vi "mobileyelanepaser3.vi"(8 "thresh  c":dbl, 9 "thresh  b":dbl, 11 "thresh r":dbl) -> (0 "cr2":dbl=0.017, 1 "cr":dbl=1.4, 2 "cl2":dbl=0.017, 3 "cl":dbl=-1.5000000000000002)   [LabVIEW 2015]
uses:
  G_LCM.vi
  G_SEN.vi
panel:
  out "cr_old":dbl
  out "cl_old":dbl
  out "r_old":dbl
  out "t0":i64
  out "b_old":dbl
  out "a2":dbl
  out "b2":dbl=0.017
  out "r2":dbl
  in  "a_cut":dbl=0.01
  out "appended array 2":bool[](array[boolean])=[TRUE, TRUE, FALSE, TRUE, TRUE, FALSE, TRUE]
  out "appended array":dbl[](array[numeric])=[0.65, 0.000478076055664682, 0.04157183092736362, 1.1538500967845816e-15]
  in  "path_gain":dbl=0.95
  in  "q_cut":dbl=0.5
  in  "dc_cut":dbl=0.55
  in  "db_cut":dbl=0.042
  in  "da_cut":dbl=0.0045
  out "lane_old":dbl[](array[numeric])=[0.0006866761302459269, 1.5821018040866166e-06, -1.3046846474672603e-05, 0.0001716690325614815]
  in  "gain":dbl=1.0
  out "dt":dbl=0.096219
  out "count":u64
  out "lane_empty":dbl[](array[numeric])
  out "Lane_R_M":dbl[](array[numeric])=[0.8, 0.0036309999999999997, 0.017, 1.4]
  out "Lane_L_M":dbl[](array[numeric])=[0.8, 0.0036309999999999997, 0.017, -1.5000000000000002]
  out "r":dbl=137.70311209033324
  in  "shift_c":dbl=-0.1
  in  "bias_b":dbl=0.005
  out "a":dbl=0.0036309999999999997
  out "b":dbl=0.017
  out "confidance_L":u8=2
  out "confidance_R":u8=2
  in  "bias_c":dbl=0.8
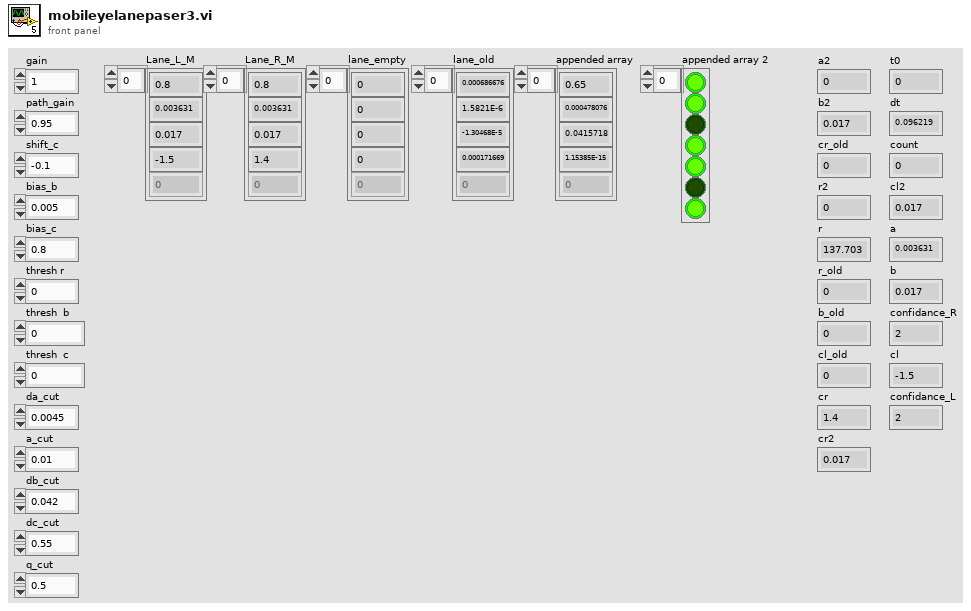
[diagram p1: front panel]
types:
  T1 = cluster{"hash":i64, "sys time":i64, "mobileye":u8[]}
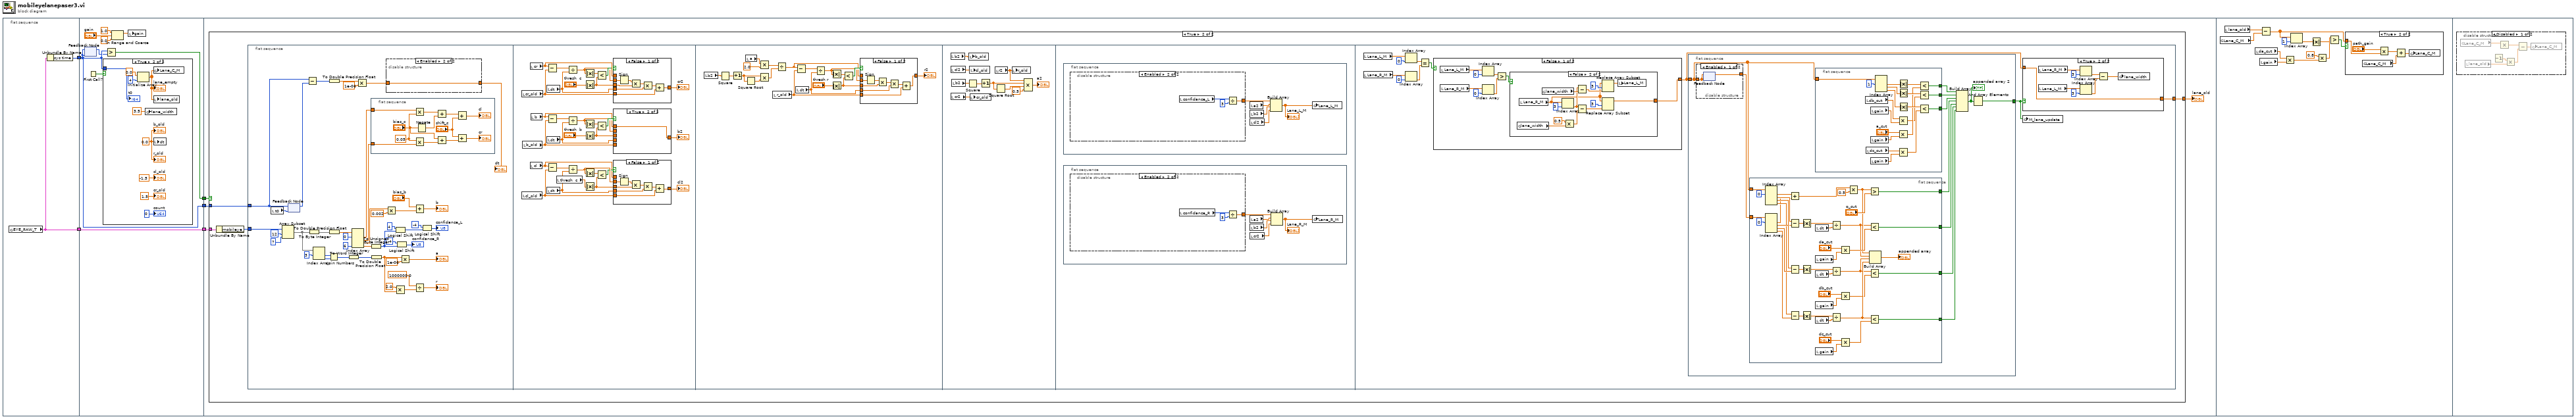
[diagram p0: block diagram]
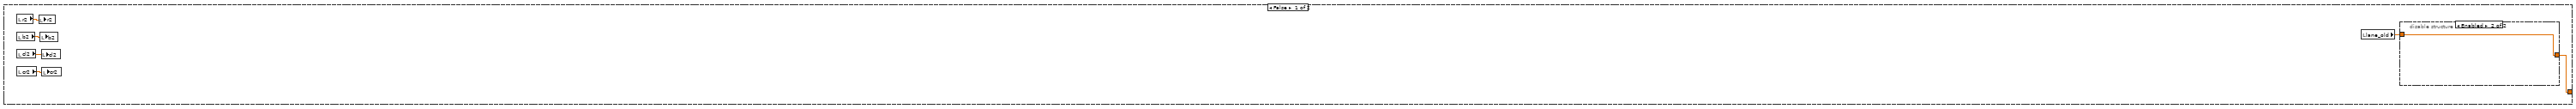
[diagram p3: hidden frame]
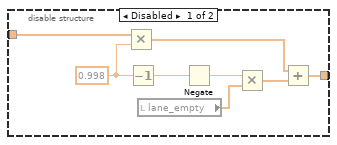
[diagram p4: hidden frame]
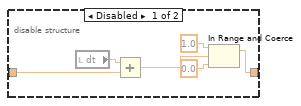
[diagram p5: hidden frame]
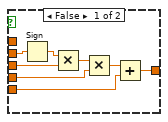
[diagram p8: hidden frame]
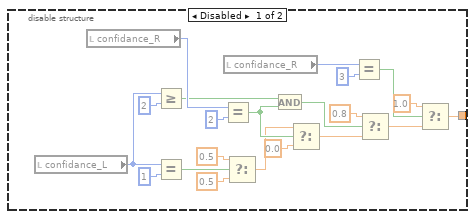
[diagram p10: hidden frame]
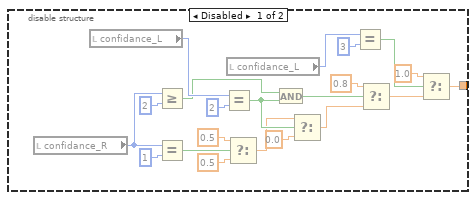
[diagram p11: hidden frame]
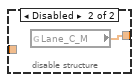
[diagram p12: hidden frame]
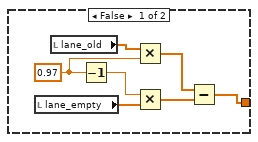
[diagram p13: hidden frame]
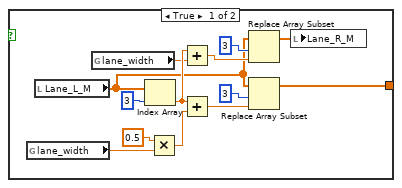
[diagram p14: hidden frame]
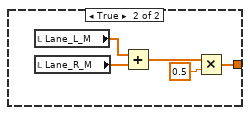
[diagram p15: hidden frame]
diagram:
  n1 = flat-sequence {
    tunnel: [w7] -> w5
    tunnel: [w6] -> w4
    tunnel: w5 -> [w16]
    tunnel: [w16] -> w3
    tunnel: w4 -> [w9]
    tunnel: [w10] -> w2
    tunnel: [w9] -> w1
    tunnel: w3 -> [w29]
    tunnel: w2 -> [w26]
    tunnel: w1 -> [w27]
    frame #0 {
      n2 = global read "G_LCM.vi" "EYE_RAW_T"() -> (w7:T1)
      n3 = Unbundle By Name(w7) -> ("sys time"=w6:i64)
    }
    frame #1 {
      n4 = feedback #1(w9) -> (w8:i64)
      n5 = feedback-in #1(w9) -> ()
      n6 = First Call?() -> (First Call?: T/F=w15:bool)
      n7 = case shown="True" w15 {
        tunnel: w9 -> [_ w20]
        frame False {
        }
        frame True {
          w19 = 0.0 ("dt2")
          n8 = Initialize Array(0.0 ("element"), 4 ("dimension size")) -> (w21:dbl[])
          "lane_empty" <- w21
          n9 = global write "G_SEN.vi" "lane_width"(3.5 ("lane_width")) -> ()
          n10 = global write "G_SEN.vi" "Lane_C_M"(w21) -> ()
          n11 = local write "lane_old"(w21) -> ()
          n12 = local write "dt"(w19) -> ()
          "count" <- u64 0
          "b_old" <- w19
          "t0" <- w20
          "r_old" <- w19
          "cl_old" <- -1.5 ("cl_old")
          "cr_old" <- 1.5 ("cr_old")
        }
      }
      n13 = Greater?(x=w9, y=w8) -> (0:w10:bool)
      n14 = In Range and Coerce(upper limit=1.0, x="gain", lower limit=0.0) -> (coerced(x)=w11:dbl)  [unwired: 1 out]
      n15 = local write "gain"(w11) -> ()
    }
    frame #2 {
      n16 = case shown="True" w26 {
        tunnel: w29 -> [_ w47]
        tunnel: [w34 w46] -> w28
        tunnel: w27 -> [_ w45]
        frame False {
          n17 = local read "r2"() -> (w33:dbl)
          n18 = local read "b2"() -> (w32:dbl)
          n19 = local read "cl2"() -> (w30:dbl)
          n20 = local read "cr2"() -> (w31:dbl)
          n21 = local write "r2"(w33) -> ()
          n22 = local write "b2"(w32) -> ()
          n23 = local write "cl2"(w30) -> ()
          n24 = local write "cr2"(w31) -> ()
          n25 = local read "lane_old"() -> (w35:dbl[])
          n26 = disable-structure shown="Enabled" {
            disable-tunnel: w35 -> [w39 w44]
            disable-tunnel: [w36 w44] -> w34
            frame Disabled {
              w38 = 0.998
              n27 = Multiply(x=w39, y=w38) -> (x*y=w42:dbl[])
              n28 = Decrement(x=w38) -> (x-1=w40:dbl)
              n29 = local read "lane_empty"() -> (w37:dbl[])
              n30 = Negate(x=w40) -> (-x=w41:dbl)
              n31 = Multiply(x=w41, y=w37) -> (x*y=w43:dbl[])
              n32 = Add(x=w42, y=w43) -> (x+y=w36:dbl[])
            }
            frame Enabled {
            }
          }
        }
        frame True {
          n33 = Unbundle By Name(w47) -> ("mobileye"=w48:u8[])
          n34 = flat-sequence {
            tunnel: w48 -> [w69]
            tunnel: w45 -> [w51]
            tunnel: [w264] -> w46
            frame #0 {
              n35 = local read "t0"() -> (w50:i64)
              n36 = Array Subset(array=w69, index=12, length=7) -> (w68:u8[])
              n37 = feedback #2(w50) -> (w52:i64)
              n38 = feedback-in #2(w51) -> ()
              n39 = Subtract(x=w51, y=w52) -> (x-y=w53:i64)
              n40 = To Byte Integer(number=w68) -> (8bit integer=w88:i8[])
              n41 = Index Array(array=w68, index #1=3 ("index")) -> (element #1=w82:u8, element #2=w81:u8)  [unwired: 1 in]
              n42 = Join Numbers(hi=w82, lo=w81) -> ((hi.lo)=w80:u16)
              n43 = To Double Precision Float(number=w53) -> (double precision float=w57:dbl)
              n44 = To Double Precision Float(number=w88) -> (double precision float=w87:dbl[])
              n45 = To Word Integer(number=w80) -> (16bit integer=w79:i16)
              n46 = Index Array(array=w87, index #1=0 ("index"), index #4=6 ("index")) -> (element #1=w86:dbl, element #2=w85:dbl, element #3=w84:dbl, element #4=w75:dbl)  [unwired: 2 in]
              n47 = Multiply(x=w57, y=1e-06) -> (x*y=w55:dbl)
              n48 = To Unsigned Byte Integer(number=w75) -> (unsigned 8bit integer=w73:u8)
              n49 = To Double Precision Float(number=w79) -> (double precision float=w58:dbl)
              n50 = flat-sequence {
                tunnel: w86 -> [w110]
                tunnel: w85 -> [w109]
                frame #0 {
                  w108 = 0.05 ("y")
                  n51 = Multiply(x=w110, y=w108) -> (x*y=w106:dbl)
                  n52 = Multiply(x=w108, y=w109) -> (x*y=w107:dbl)
                  n53 = Negate(x="bias_c") -> (-x=w104:dbl)
                  n54 = Add(x=w106, y=w104) -> (x+y=w103:dbl)
                  n55 = Add(x="bias_c", y=w107) -> (x+y=w101:dbl)
                  n56 = Add(x=w103, y="shift_c") -> (x+y=→"cl":dbl)
                  n57 = Add(x="shift_c", y=w101) -> (x+y=→"cr":dbl)
                }
              }
              n58 = Multiply(x=w84, y=0.002) -> (x*y=w65:dbl)
              n59 = disable-structure shown="Enabled" {
                disable-tunnel: w55 -> [w97 w98]
                disable-tunnel: [w92 w98] -> w54
                frame Disabled {
                  n60 = local read "dt"() -> (w96:dbl)
                  n61 = Add(x=w96, y=w97) -> (x+y=w95:dbl)
                  n62 = In Range and Coerce(upper limit=1.0, x=w95, lower limit=0.0) -> (coerced(x)=w92:dbl)  [unwired: 1 out]
                }
                frame Enabled {
                }
              }
              "dt" <- w54
              n63 = Logical Shift(y=i16 4, x=w73) -> (x << y=w71:u8)
              n64 = Multiply(x=2.0, y=w58) -> (x*y=w61:dbl)
              n65 = Logical Shift(y=i16 -4, x=w73) -> (x << y=→"confidance_R":u8)
              n66 = Multiply(x=w58, y=1e-06) -> (x*y=→"a":dbl)
              n67 = Add(x="bias_b", y=w65) -> (x+y=→"b":dbl)
              n68 = Divide(x=1000000.0 ("y"), y=w61) -> (x/y=→"r":dbl)
              n69 = Logical Shift(y=i16 -4, x=w71) -> (x << y=→"confidance_L":u8)
            }
            frame #1 {
              n70 = local read "cr_old"() -> (w112:dbl)
              n71 = local read "cl_old"() -> (w131:dbl)
              n72 = local read "b_old"() -> (w132:dbl)
              n73 = local read "cr"() -> (w121:dbl)
              n74 = local read "cl"() -> (w123:dbl)
              n75 = local read "b"() -> (w122:dbl)
              n76 = Subtract(x=w121, y=w112) -> (x-y=w119:dbl)
              n77 = Subtract(x=w122, y=w132) -> (x-y=w139:dbl)
              n78 = Subtract(x=w123, y=w131) -> (x-y=w125:dbl)
              n79 = local read "dt"() -> (w113:dbl)
              n80 = local read "dt"() -> (w133:dbl)
              n81 = local read "dt"() -> (w130:dbl)
              n82 = local read "thresh  c"() -> (w111:dbl)
              n83 = Divide(x=w119, y=w113) -> (x/y=w115:dbl)
              n84 = Divide(x=w139, y=w133) -> (x/y=w135:dbl)
              n85 = Divide(x=w125, y=w130) -> (x/y=w128:dbl)
              n86 = Absolute Value(x=w115) -> (abs(x)=w118:dbl)
              n87 = Absolute Value(x="thresh  c") -> (abs(x)=w114:dbl)
              n88 = Absolute Value(x=w135) -> (abs(x)=w138:dbl)
              n89 = Absolute Value(x="thresh  b") -> (abs(x)=w134:dbl)
              n90 = Absolute Value(x=w128) -> (abs(x)=w126:dbl)
              n91 = Absolute Value(x=w111) -> (abs(x)=w129:dbl)
              n92 = Less?(x=w118, y=w114) -> (x < y?=w117:bool)
              n93 = Less?(x=w138, y=w134) -> (x < y?=w137:bool)
              n94 = Less?(x=w126, y=w129) -> (x < y?=w127:bool)
              n95 = case shown="False" w117 {
                tunnel: [w147 w149] -> w120
                tunnel: w115 -> [w145 _]
                tunnel: w114 -> [w144 _]
                tunnel: w113 -> [w142 _]
                tunnel: w112 -> [w141 _]
                tunnel: w121 -> [_ w149]
                frame False {
                  n96 = Sign(1:w145) -> (0:w143:dbl)
                  n97 = Multiply(x=w143, y=w144) -> (x*y=w148:dbl)
                  n98 = Multiply(x=w148, y=w142) -> (x*y=w146:dbl)
                  n99 = Add(x=w146, y=w141) -> (x+y=w147:dbl)
                }
                frame True {
                }
              }
              "cr2" <- w120
              n100 = case shown="True" w137 {
                tunnel: [w165 w167] -> w140
                tunnel: w135 -> [w163 _]
                tunnel: w134 -> [w162 _]
                tunnel: w133 -> [w160 _]
                tunnel: w132 -> [w159 _]
                tunnel: w122 -> [_ w167]
                frame False {
                  n101 = Sign(1:w163) -> (0:w161:dbl)
                  n102 = Multiply(x=w161, y=w162) -> (x*y=w166:dbl)
                  n103 = Multiply(x=w166, y=w160) -> (x*y=w164:dbl)
                  n104 = Add(x=w164, y=w159) -> (x+y=w165:dbl)
                }
                frame True {
                }
              }
              "b2" <- w140
              n105 = case shown="False" w127 {
                tunnel: [w156 w158] -> w124
                tunnel: w128 -> [w154 _]
                tunnel: w129 -> [w153 _]
                tunnel: w130 -> [w151 _]
                tunnel: w131 -> [w150 _]
                tunnel: w123 -> [_ w158]
                frame False {
                  n106 = Sign(1:w154) -> (0:w152:dbl)
                  n107 = Multiply(x=w152, y=w153) -> (x*y=w157:dbl)
                  n108 = Multiply(x=w157, y=w151) -> (x*y=w155:dbl)
                  n109 = Add(x=w155, y=w150) -> (x+y=w156:dbl)
                }
                frame True {
                }
              }
              "cl2" <- w124
            }
            frame #2 {
              n110 = local read "b2"() -> (w173:dbl)
              n111 = Square(x=w173) -> (x^2=w174:dbl)
              n112 = Increment(x=w174) -> (x+1=w176:dbl)
              n113 = Square Root(x=w176) -> (sqrt(x)=w175:dbl)
              n114 = local read "a"() -> (w170:dbl)
              n115 = Multiply(x=w170, y=2.0) -> (x*y=w172:dbl)
              n116 = Multiply(x=w176, y=w175) -> (x*y=w177:dbl)
              n117 = local read "r_old"() -> (w168:dbl)
              n118 = Divide(x=w172, y=w177) -> (x/y=w178:dbl)
              n119 = Subtract(x=w178, y=w168) -> (x-y=w185:dbl)
              n120 = local read "dt"() -> (w169:dbl)
              n121 = Divide(x=w185, y=w169) -> (x/y=w180:dbl)
              n122 = Absolute Value(x=w180) -> (abs(x)=w184:dbl)
              n123 = Absolute Value(x="thresh r") -> (abs(x)=w179:dbl)
              n124 = Less?(x=w184, y=w179) -> (x < y?=w183:bool)
              n125 = case shown="False" w183 {
                tunnel: [w192 w194] -> w182
                tunnel: w180 -> [w190 _]
                tunnel: w179 -> [w189 _]
                tunnel: w169 -> [w187 _]
                tunnel: w178 -> [_ w194]
                tunnel: w168 -> [w186 _]
                frame False {
                  n126 = Sign(1:w190) -> (0:w188:dbl)
                  n127 = Multiply(x=w188, y=w189) -> (x*y=w193:dbl)
                  n128 = Multiply(x=w193, y=w187) -> (x*y=w191:dbl)
                  n129 = Add(x=w191, y=w186) -> (x+y=w192:dbl)
                }
                frame True {
                }
              }
              "r2" <- w182
            }
            frame #3 {
              n130 = local read "b2"() -> (w198:dbl)
              n131 = local read "cl2"() -> (w196:dbl)
              n132 = local read "cr2"() -> (w195:dbl)
              n133 = local read "b2"() -> (w204:dbl)
              n134 = Square(x=w204) -> (x^2=w203:dbl)
              n135 = local write "b_old"(w198) -> ()
              n136 = local write "cl_old"(w196) -> ()
              n137 = local write "cr_old"(w195) -> ()
              n138 = Increment(x=w203) -> (x+1=w201:dbl)
              n139 = local read "r2"() -> (w197:dbl)
              n140 = Square Root(x=w201) -> (sqrt(x)=w202:dbl)
              n141 = local write "r_old"(w197) -> ()
              n142 = Compound Arithmetic op=MULTIPLY(w197, w201, w202, 0.5 ("value")) -> (→"a2":dbl)
            }
            frame #4 {
              n143 = flat-sequence {
                frame #0 {
                  n144 = disable-structure shown="Enabled" {
                    disable-tunnel: [w256 w260] -> w235
                    frame Disabled {
                      n145 = local read "confidance_R"() -> (w244:u8)
                      n146 = local read "confidance_L"() -> (w250:u8)
                      n147 = Greater Or Equal?(x=w244, y=u8 2) -> (x >= y?=w246:bool)
                      n148 = Equal?(x=w244, y=u8 1) -> (x = y?=w242:bool)
                      n149 = Equal?(x=w250, y=u8 2) -> (x = y?=w245:bool)
                      n150 = local read "confidance_L"() -> (w257:u8)
                      n151 = Select(t=0.5, s=w242, f=0.5 ("t")) -> (s? t:f=w239:dbl)
                      n152 = And(x=w246, y=w245) -> (x .and. y?=w253:bool)
                      n153 = Select(t=w239, s=w245, f=0.0) -> (s? t:f=w248:dbl)
                      n154 = Equal?(x=w257, y=u8 3) -> (x = y?=w254:bool)
                      n155 = Select(t=0.8, s=w253, f=w248) -> (s? t:f=w251:dbl)
                      n156 = Select(t=1.0, s=w254, f=w251) -> (s? t:f=w256:dbl)
                    }
                    frame Enabled {
                      n157 = local read "confidance_L"() -> (w262:u8)
                      n158 = Divide(x=w262, y=u8 3) -> (x/y=w260:dbl)
                    }
                  }
                  n159 = local read "a2"() -> (w236:dbl)
                  n160 = local read "b2"() -> (w237:dbl)
                  n161 = local read "cl2"() -> (w238:dbl)
                  n162 = Build Array(w235, w236, w237, w238) -> (w234:dbl[])
                  "Lane_L_M" <- w234
                  n163 = global write "G_SEN.vi" "Lane_L_M"(w234) -> ()
                }
              }
              n164 = flat-sequence {
                frame #0 {
                  n165 = disable-structure shown="Enabled" {
                    disable-tunnel: [w227 w231] -> w206
                    frame Disabled {
                      n166 = local read "confidance_L"() -> (w210:u8)
                      n167 = local read "confidance_R"() -> (w221:u8)
                      n168 = Greater Or Equal?(x=w210, y=u8 2) -> (x >= y?=w217:bool)
                      n169 = Equal?(x=w210, y=u8 1) -> (x = y?=w213:bool)
                      n170 = Equal?(x=w221, y=u8 2) -> (x = y?=w216:bool)
                      n171 = local read "confidance_R"() -> (w228:u8)
                      n172 = Select(t=0.5, s=w213, f=0.5 ("t")) -> (s? t:f=w211:dbl)
                      n173 = And(x=w217, y=w216) -> (x .and. y?=w224:bool)
                      n174 = Select(t=w211, s=w216, f=0.0) -> (s? t:f=w218:dbl)
                      n175 = Equal?(x=w228, y=u8 3) -> (x = y?=w226:bool)
                      n176 = Select(t=0.8, s=w224, f=w218) -> (s? t:f=w222:dbl)
                      n177 = Select(t=1.0, s=w226, f=w222) -> (s? t:f=w227:dbl)
                    }
                    frame Enabled {
                      n178 = local read "confidance_R"() -> (w232:u8)
                      n179 = Divide(x=w232, y=u8 3) -> (x/y=w231:dbl)
                    }
                  }
                  n180 = local read "a2"() -> (w207:dbl)
                  n181 = local read "b2"() -> (w208:dbl)
                  n182 = local read "cr2"() -> (w209:dbl)
                  n183 = Build Array(w206, w207, w208, w209) -> (w205:dbl[])
                  "Lane_R_M" <- w205
                  n184 = global write "G_SEN.vi" "Lane_R_M"(w205) -> ()
                }
              }
            }
            frame #5 {
              n185 = local read "Lane_L_M"() -> (w265:dbl[])
              n186 = local read "Lane_R_M"() -> (w266:dbl[])
              n187 = Index Array(array=w265, index=0) -> (element=w270:dbl)
              n188 = Index Array(array=w266, index=0) -> (element=w269:dbl)
              n189 = Equal?(x=w270, y=w269) -> (x = y?=w268:bool)
              n190 = case shown="False" w268 {
                tunnel: [w366 w400] -> w267
                frame False {
                  n191 = local read "Lane_L_M"() -> (w364:dbl[])
                  n192 = local read "Lane_R_M"() -> (w365:dbl[])
                  n193 = Index Array(array=w364, index=0) -> (element=w369:dbl)
                  n194 = Index Array(array=w365, index=0) -> (element=w368:dbl)
                  n195 = Greater?(x=w369, y=w368) -> (0:w367:bool)
                  n196 = case shown="False" w367 {
                    tunnel: [w381 w394] -> w366
                    frame True {
                      n197 = global read "G_SEN.vi" "lane_width"() -> (w378:dbl)
                      n198 = local read "Lane_L_M"() -> (w372:dbl[])
                      n199 = global read "G_SEN.vi" "lane_width"() -> (w374:dbl)
                      n200 = Index Array(array=w372, index=3) -> (element=w375:dbl)
                      n201 = Multiply(x=0.5 ("y"), y=w378) -> (x*y=w380:dbl)
                      n202 = Add(x=w375, y=w374) -> (x+y=w376:dbl)
                      n203 = Add(x=w375, y=w380) -> (x+y=w383:dbl)
                      n204 = Replace Array Subset(array=w372, new element=w376, index=3) -> (w373:dbl[])
                      n205 = Replace Array Subset(array=w372, new element=w383, index=3) -> (w381:dbl[])
                      n206 = local write "Lane_R_M"(w373) -> ()
                    }
                    frame False {
                      n207 = global read "G_SEN.vi" "lane_width"() -> (w391:dbl)
                      n208 = local read "Lane_R_M"() -> (w386:dbl[])
                      n209 = global read "G_SEN.vi" "lane_width"() -> (w388:dbl)
                      n210 = Index Array(array=w386, index=3) -> (element=w387:dbl)
                      n211 = Multiply(x=0.5 ("y"), y=w391) -> (x*y=w393:dbl)
                      n212 = Subtract(x=w387, y=w388) -> (x-y=w389:dbl)
                      n213 = Subtract(x=w387, y=w393) -> (x-y=w396:dbl)
                      n214 = Replace Array Subset(array=w386, new element=w389, index=3) -> (w385:dbl[])
                      n215 = Replace Array Subset(array=w386, new element=w396, index=3) -> (w394:dbl[])
                      n216 = local write "Lane_L_M"(w385) -> ()
                    }
                  }
                }
                frame True {
                  n217 = local read "Lane_L_M"() -> (w398:dbl[])
                  n218 = local read "Lane_R_M"() -> (w399:dbl[])
                  n219 = Add(x=w398, y=w399) -> (x+y=w402:dbl[])
                  n220 = Multiply(x=w402, y=0.5) -> (x*y=w400:dbl[])
                }
              }
              n221 = flat-sequence {
                tunnel: w267 -> [w280]
                tunnel: [w281] -> w263
                frame #0 {
                  n222 = disable-structure shown="Enabled" {
                    disable-tunnel: w280 -> [w347 _]
                    disable-tunnel: [w346 w348] -> w283
                    frame Enabled {
                      n223 = feedback #3(w347) -> (w346:dbl[])
                      n224 = feedback-in #3(w347) -> ()
                    }
                    frame Disabled {
                      n225 = global read "G_SEN.vi" "Lane_C_M"() -> (w348:dbl[])
                    }
                  }
                  n226 = flat-sequence {
                    tunnel: w283 -> [w311]
                    tunnel: [w303] -> w277
                    tunnel: [w302] -> w273
                    tunnel: w280 -> [w301]
                    tunnel: [w292] -> w274
                    tunnel: [w284] -> w276
                    frame #0 {
                      n227 = Index Array(array=w301, index #1=0 ("index")) -> (element #1=w297:dbl, element #2=w318:dbl, element #3=w323:dbl, element #4=w312:dbl)  [unwired: 3 in]
                      n228 = Index Array(array=w311, index #1=0 ("index")) -> (element #1=w296:dbl, element #2=w317:dbl, element #3=w322:dbl, element #4=w316:dbl)  [unwired: 3 in]
                      n229 = Add(x=w297, y=w296) -> (x+y=w295:dbl)
                      n230 = Subtract(x=w318, y=w317) -> (x-y=w325:dbl)
                      n231 = Subtract(x=w323, y=w322) -> (x-y=w319:dbl)
                      n232 = Subtract(x=w312, y=w316) -> (x-y=w313:dbl)
                      n233 = Absolute Value(x=w325) -> (abs(x)=w290:dbl)
                      n234 = Absolute Value(x=w319) -> (abs(x)=w320:dbl)
                      n235 = Absolute Value(x=w313) -> (abs(x)=w315:dbl)
                      n236 = local read "dt"() -> (w324:dbl)
                      n237 = local read "gain"() -> (w310:dbl)
                      n238 = local read "dt"() -> (w321:dbl)
                      n239 = local read "gain"() -> (w308:dbl)
                      n240 = local read "dt"() -> (w314:dbl)
                      n241 = local read "gain"() -> (w305:dbl)
                      n242 = Divide(x=w290, y=w324) -> (x/y=w289:dbl)
                      n243 = Divide(x=w320, y=w321) -> (x/y=w285:dbl)
                      n244 = Divide(x=w315, y=w314) -> (x/y=w287:dbl)
                      n245 = Multiply(x="da_cut", y=w310) -> (x*y=w304:dbl)
                      n246 = Multiply(x="db_cut", y=w308) -> (x*y=w286:dbl)
                      n247 = Multiply(x="dc_cut", y=w305) -> (x*y=w300:dbl)
                      n248 = Multiply(x=w295, y=0.5) -> (x*y=w291:dbl)
                      n249 = Greater?(x=w291, y="q_cut") -> (0:w292:bool)
                      n250 = Less?(x=w289, y=w304) -> (x < y?=w303:bool)
                      n251 = Less?(x=w285, y=w286) -> (x < y?=w284:bool)
                      n252 = Less?(x=w287, y=w300) -> (x < y?=w302:bool)
                      n253 = Build Array(w291, w289, w285, w287) -> (→"appended array":dbl[])
                    }
                  }
                  n254 = flat-sequence {
                    tunnel: w280 -> [w345]
                    tunnel: [w344] -> w278
                    tunnel: [w342] -> w275
                    tunnel: [w333] -> w279
                    frame #0 {
                      n255 = local read "db_cut"() -> (w328:dbl)
                      n256 = local read "dc_cut"() -> (w338:dbl)
                      n257 = local read "gain"() -> (w327:dbl)
                      n258 = local read "gain"() -> (w330:dbl)
                      n259 = local read "gain"() -> (w337:dbl)
                      n260 = Index Array(array=w345, index #1=1 ("index")) -> (element #1=w341:dbl, element #2=w334:dbl, element #3=w332:dbl)  [unwired: 2 in]
                      n261 = Multiply(x=w328, y=w327) -> (x*y=w326:dbl)
                      n262 = Multiply(x="a_cut", y=w330) -> (x*y=w329:dbl)
                      n263 = Multiply(x=w338, y=w337) -> (x*y=w336:dbl)
                      n264 = Absolute Value(x=w341) -> (abs(x)=w340:dbl)
                      n265 = Absolute Value(x=w334) -> (abs(x)=w335:dbl)
                      n266 = Absolute Value(x=w332) -> (abs(x)=w339:dbl)
                      n267 = Less?(x=w340, y=w329) -> (x < y?=w342:bool)
                      n268 = Less?(x=w335, y=w326) -> (x < y?=w333:bool)
                      n269 = Less?(x=w339, y=w336) -> (x < y?=w344:bool)
                    }
                  }
                  n270 = Build Array(w275, w279, w278, w274, w277, w276, w273) -> (w282:bool[])
                  "appended array 2" <- w282
                  n271 = And Array Elements(Boolean array=w282) -> (logical AND=w281:bool)
                }
              }
              n272 = case shown="True" w263 {
                tunnel: w267 -> [_ w356]
                tunnel: [w350 w356] -> w264
                frame False {
                  w352 = 0.97
                  n273 = local read "lane_empty"() -> (w351:dbl[])
                  n274 = local read "lane_old"() -> (w353:dbl[])
                  n275 = Decrement(x=w352) -> (x-1=w349:dbl)
                  n276 = Multiply(x=w353, y=w352) -> (x*y=w354:dbl[])
                  n277 = Multiply(x=w349, y=w351) -> (x*y=w355:dbl[])
                  n278 = Subtract(x=w354, y=w355) -> (x-y=w350:dbl[])
                }
                frame True {
                  n279 = local read "Lane_R_M"() -> (w358:dbl[])
                  n280 = local read "Lane_L_M"() -> (w357:dbl[])
                  n281 = Index Array(array=w358, index=3) -> (element=w362:dbl)
                  n282 = Index Array(array=w357, index=3) -> (element=w361:dbl)
                  n283 = Subtract(x=w362, y=w361) -> (x-y=w360:dbl)
                  n284 = global write "G_SEN.vi" "lane_width"(w360) -> ()
                }
              }
              n285 = global write "G_SEN.vi" "M_lane_update"(w263) -> ()
            }
          }
        }
      }
      "lane_old" <- w28
    }
    frame #3 {
      n286 = global read "G_SEN.vi" "Lane_C_M"() -> (w413:dbl[])
      n287 = local read "lane_old"() -> (w414:dbl[])
      n288 = local read "da_cut"() -> (w408:dbl)
      n289 = local read "gain"() -> (w409:dbl)
      n290 = Subtract(x=w414, y=w413) -> (x-y=w412:dbl[])
      n291 = Multiply(x=w408, y=w409) -> (x*y=w404:dbl)
      n292 = Index Array(array=w412, index=1) -> (element=w410:dbl)
      n293 = Absolute Value(x=w410) -> (abs(x)=w406:dbl)
      n294 = Multiply(x=0.8, y=w404) -> (x*y=w407:dbl)
      n295 = Greater?(x=w407, y=w406) -> (0:w405:bool)
      n296 = case shown="True" w405 {
        tunnel: w412 -> [_ w415]
        frame False {
        }
        frame True {
          n297 = global read "G_SEN.vi" "Lane_C_M"() -> (w419:dbl[])
          n298 = Multiply(x="path_gain", y=w415) -> (x*y=w416:dbl[])
          n299 = Add(x=w416, y=w419) -> (x+y=w418:dbl[])
          n300 = global write "G_SEN.vi" "Lane_C_M"(w418) -> ()
        }
      }
    }
    frame #4 {
      n301 = disable-structure shown="Disabled" {
        frame Disabled {
          n302 = global read "G_SEN.vi" "Lane_C_M"() -> (w425:dbl[])
          n303 = local read "lane_old"() -> (w421:dbl[])
          n304 = Decrement() -> (x-1=w420:dbl)  [unwired: 1 in]
          n305 = Multiply(x=w425) -> (x*y=w424:dbl[])  [unwired: 1 in]
          n306 = Multiply(x=w420, y=w421) -> (x*y=w423:dbl[])
          n307 = Subtract(x=w424, y=w423) -> (x-y=w422:dbl[])
          n308 = global write "G_SEN.vi" "Lane_C_M"(w422) -> ()
        }
        frame Enabled {
        }
      }
    }
  }
